vi "Write Color.vi"(8 "error in (no error)":errorcluster, 10 "Color in":u32(colorbox), 11 "RectangleShape in":refnum<class "RectangleShape.lvclass">) -> (0 "error out":errorcluster, 3 "RectangleShape out":refnum<class "RectangleShape.lvclass">)   [LabVIEW 2022 SP3, in "RectangleShape.lvclass"]
uses:
  RectangleShape.lvclass
  RectangleShape.lvclass/RectangleShape.ctl
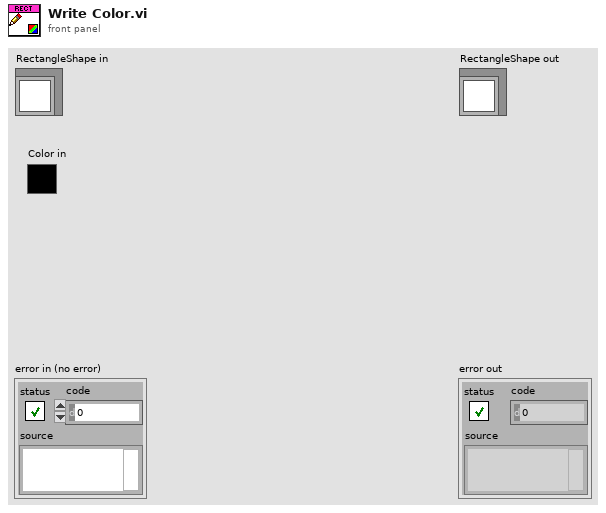
[diagram p1: front panel]
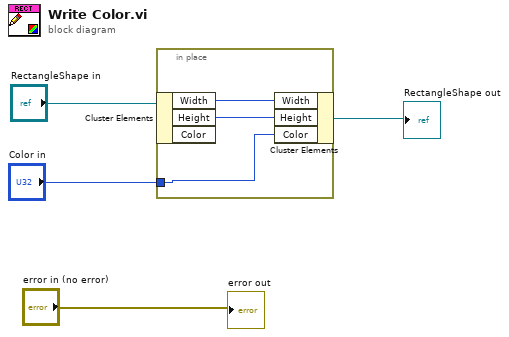
[diagram p0: block diagram]
diagram:
  n1 = in-place {
    in-place-border: "Color in" -> [w5]
    n2 = in-place-cluster #1("RectangleShape in") -> ("Width"=w7:i16, "Height"=w6:i16)  [unwired: 1 out]
    n3 = in-place-cluster #1("Width"=w7, "Height"=w6, "Color"=w5) -> (→"RectangleShape out":refnum<class "RectangleShape.lvclass">)
  }
  "error out" <- "error in (no error)"
